vi "Test Performance.vi"() -> ()   [LabVIEW 2019]
uses:
  <vilib>/Analysis/baseanly.llb/Mean (DBL).vi
  src/subVIs/Circular Buffer (waveform).vi
  src/xy_utilities.lvlib
  <vilib>/Analysis/NI_AALBase.lvlib
  <vilib>/measure/NI_MABase.lvlib
panel:
  out "XY Data 3":cluster{"X-array":dbl[], "Y-array":dbl[]}[](graph)
  out "Intensity Graph 2":dbl[][](graph)
  out "Intensity Graph":dbl[][](graph)
  out "execution time (s)":dbl format="%#_6p"
  out "XY Data 2":cluster{"X-array":dbl[], "Y-array":dbl[]}(graph)
  out "XY Data":cluster{"X-array":dbl[], "Y-array":dbl[]}[](graph)
  # "0: 21\"\n5: 0.09\""
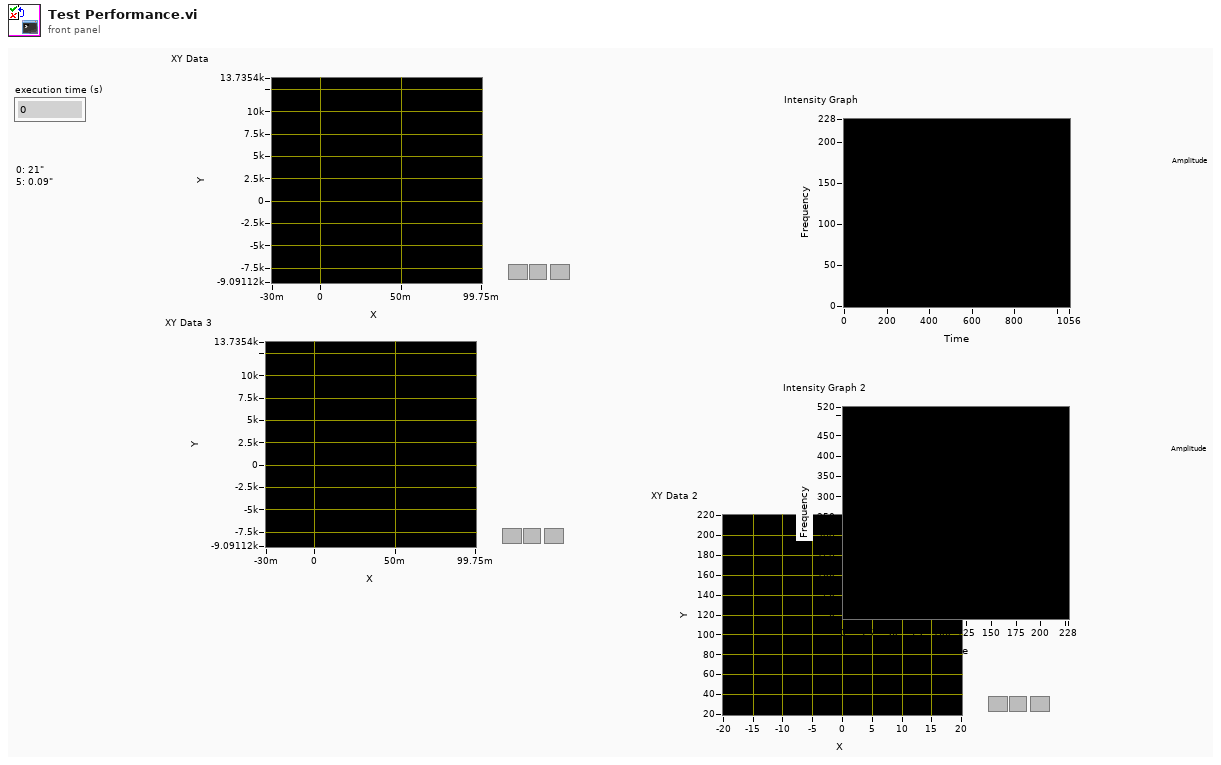
[diagram p1: front panel]
types:
  T1 = enum16{"thermal waveguide", "superlattice waveguide", "decay in atmosphere"}
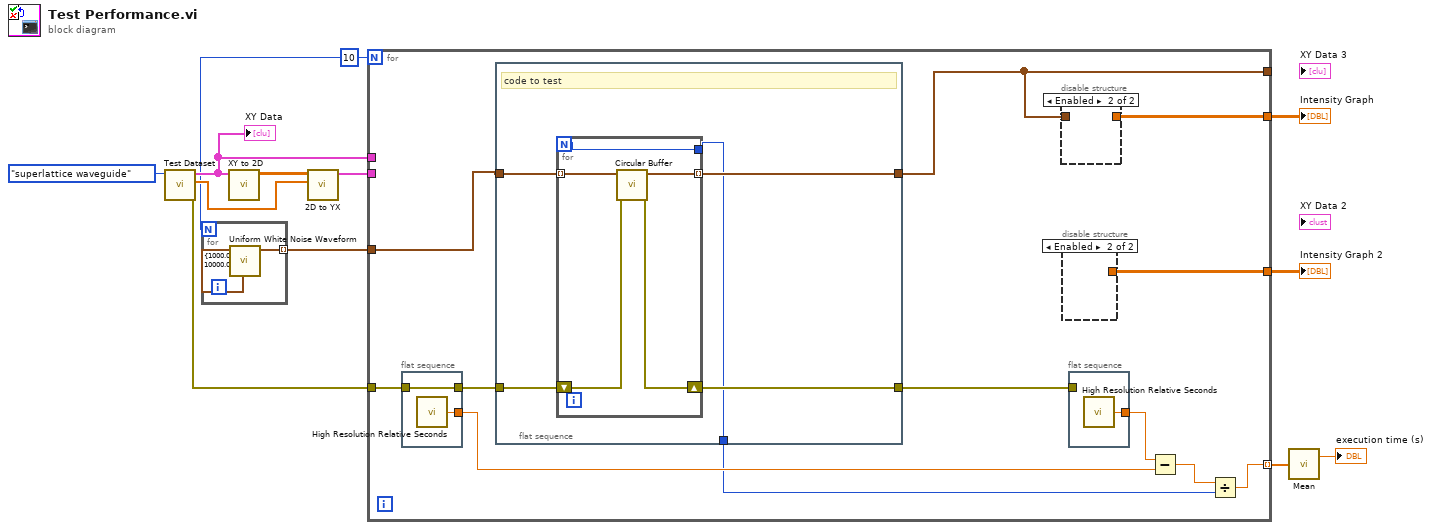
[diagram p0: block diagram]
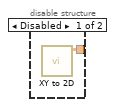
[diagram p2: hidden frame]
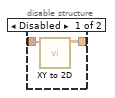
[diagram p3: hidden frame]
diagram:
  w1 = 10
  n1 = call "Test Dataset.vi"("Enum"=T1."superlattice waveguide") -> ("error out"=w12:errorcluster, "Parameters out"=w7:dbl[], "XY-data out"=w4:cluster{"X-array":dbl[], "Y-array":dbl[]}[])  [unwired: 8 in]
  "XY Data" <- w4
  n2 = for {
    N: w1 -> [_]
    tunnel: [w14] -> w2 mode=indexing
    n3 = call <vilib>:"Uniform White Noise Waveform.vi"("sampling info"=cluster{"Fs":dbl, "#s":dbl} {"Fs"=1000.0, "#s"=10000.0}) -> ("signal out"=w14:waveform(dbl))  [unwired: 9 in, 1 out]
  }
  n4 = call "XY to 2D.vi"("XY-data"=w4) -> ("2D Z Array"=w6:dbl[][])  [unwired: 7 in, 3 out]
  n5 = call "2D to YX.vi"("Y Array"=w7, "2D Z Array"=w6) -> ("XY-data out"=w5:cluster{"X-array":dbl[], "Y-array":dbl[]}[])  [unwired: 8 in, 1 out]
  n6 = for {
    N: w1 -> [_]
    tunnel: w12 -> [w26]
    tunnel: w5 -> [_]
    tunnel: [w23] -> w11
    tunnel: [w22] -> w10
    tunnel: [w16] -> w8 mode=indexing
    tunnel: [w19] -> _
    tunnel: w4 -> [_]
    tunnel: w2 -> [w15]
    n7 = flat-sequence {
      tunnel: [w42] -> w21
      tunnel: w26 -> [w42]
      tunnel: [w41] -> w24
      frame #0 {
        n8 = call <vilib>:"High Resolution Relative Seconds.vi"() -> ("relative seconds"=w41:dbl)
      }
    }
    n9 = flat-sequence {
      tunnel: w15 -> [w34]
      tunnel: w21 -> [w32]
      tunnel: [w31] -> w20
      tunnel: [w33] -> w19
      tunnel: [w30] -> w18
      frame #0 {
        # "code to test"
        n10 = for {
          N -> [w35]
          tunnel: w34 -> [w39] mode=indexing
          tunnel: [w38] -> w33 mode=indexing
          shift-right: [w36] -> w31
          shift-left: w32 -> [w37]
          tunnel: [w35] -> w30
          n11 = call-poly "Circular Buffer.vi"("error in"=w37, "Waveform in"=w39) -> ("error out"=w36:errorcluster, "Waveform out"=w38:waveform(dbl))  [unwired: 8 in]
        }
      }
    }
    n12 = disable-structure shown="Enabled" {
      disable-tunnel: [w29 _] -> w22
      disable-tunnel: w19 -> [w28 _]
      frame Disabled {
        n13 = call "XY to 2D.vi"("XY-data"=w28) -> ("2D Z Array"=w29:dbl[][])  [unwired: 7 in, 3 out]
      }
      frame Enabled {
      }
    }
    n14 = disable-structure shown="Enabled" {
      disable-tunnel: [w27 _] -> w23
      frame Disabled {
        n15 = call "XY to 2D.vi"() -> ("2D Z Array"=w27:dbl[][])  [unwired: 8 in, 3 out]
      }
      frame Enabled {
      }
    }
    n16 = flat-sequence {
      tunnel: [w40] -> w25
      tunnel: w20 -> [_]
      frame #0 {
        n17 = call <vilib>:"High Resolution Relative Seconds.vi"() -> ("relative seconds"=w40:dbl)
      }
    }
    n18 = Subtract(x=w25, y=w24) -> (x-y=w17:dbl)
    n19 = Divide(x=w17, y=w18) -> (x/y=w16:dbl)
  }
  "Intensity Graph" <- w10
  "Intensity Graph 2" <- w11
  n20 = call-poly <vilib>:"Mean.vi"("X"=w8) -> ("mean"=→"execution time (s)":dbl)  [unwired: 1 out]
